vi "0x2 RIO-OCU update.vi"(11 "NetworkStreamWriter In":refnum<class "NetworkStreamWriter.lvclass">) -> (3 "NetworkStreamWriter Out":refnum<class "NetworkStreamWriter.lvclass">)   [LabVIEW 2011]
doc: "Sends general data up to the listening OCU over a network stream for monitoring and debugging purposes."
uses:
  0x2 Typedefs/RIO-OCU update controls.ctl
  2-Think/2 Typedefs/generalized sensor status.ctl
  2-Think/2 Typedefs/indicator LED.ctl
  2-Think/2 Typedefs/generalized actuator status.ctl
  2-Think/2 Typedefs/Which Boat.ctl
  2-Think/2 Typedefs/robot velocity.ctl
  2-Think/2 Typedefs/UTM Location.ctl
  2-Think/2 Typedefs/heading.ctl
  2-Think/2 Typedefs/rate of turn.ctl
  2-Think/2 Typedefs/pitch and roll.ctl
  2-Think/2 Typedefs/apparent wind.ctl
  2-Think/2 Typedefs/apparent wind speed.ctl
  2-Think/2 Typedefs/apparent wind direction.ctl
  2-Think/2 Typedefs/Velocity.ctl
  2-Think/2 Typedefs/absolute wind direction.ctl
  2-Think/2 Typedefs/absolute wind speed.ctl
  2-Think/2 Typedefs/absolute water current vector.ctl
  2-Think/2 Typedefs/rudder angle.ctl
  2-Think/2 Typedefs/sail setpt.ctl
  2-Think/2 Typedefs/manual override.ctl
  2-Think/2 Typedefs/setpoints to boat.ctl
  0x2 Typedefs/Waypoints List.ctl
  0x2 Typedefs/ocuWaypoint.ctl
  0x2 Typedefs/waypointTypes.ctl
  0x2 Typedefs/Current Waypoint.ctl
  0x2 Classes/NetworkStreams/Writer/NetworkStreamWriter.lvclass
  2-Think/2 Globals/2 Global.vi
panel:
  out "RIO->OCU update data":T1 {"Robot Pitch/Roll"."Roll" format="%05.1f"; "Robot Pitch/Roll"."Pitch" format="%05.1f"; "Robot\nRate of Turn" format="%05.1f"; "Robot\nHeading" format="%05.1f"}
  # "How Am I?"
  # "Where Am I?"
  # "Path Planning"
  # "From Planning Functions"
  # "(this is not a cluster because subitems\nare generated in parallel code)"
  # "What's Around Me?"
  # "As Measured"
  # "As Measured"
  # "Loop Rates"
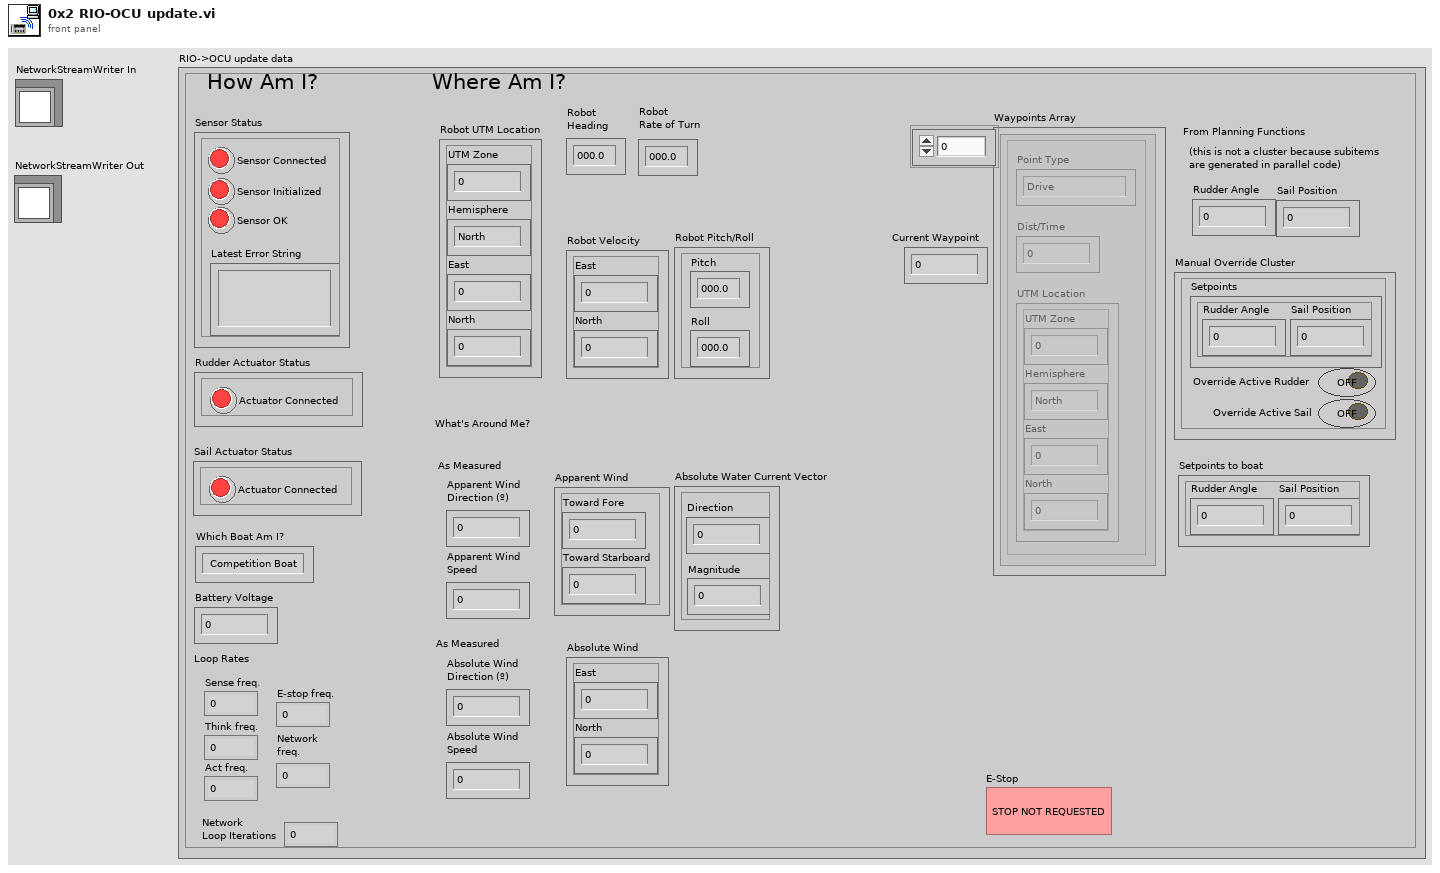
[diagram p1: front panel]
types:
  T1 = typedef "RIO-OCU update controls.ctl" = cluster{"Sensor Status":T2, "Battery Voltage":dbl, "Rudder Actuator Status":T4, "Sail Actuator Status":T4, "Which Boat Am I?":T5, "Robot Velocity":T6, "Robot UTM Location":T7, "Robot\nHeading ":T8, "Robot\nRate of Turn":T9, "Robot Pitch/Roll":T10, "Apparent Wind":T11, "Apparent Wind\nSpeed":T12, "Apparent Wind\nDirection (º)":T13, "Absolute Wind":T14, "Absolute Wind\nDirection (º)":T15, "Absolute Wind\nSpeed":T16, "Absolute Water Current Vector":T17, "Rudder Angle":T18, "Sail Position":T19, "Manual Override Cluster":T20, "Setpoints to boat":T21, "Waypoints Array":T22, "Current Waypoint":T25, "Think freq.":dbl, "Sense freq.":dbl, "Act freq.":dbl, "E-stop freq.":dbl, "Network \nfreq.":dbl, "Network \nLoop Iterations":i64, "E-Stop":bool}
  T2 = typedef "generalized sensor status.ctl" = cluster{"Sensor Connected":T3, "Sensor Initialized":T3, "Sensor OK":T3, "Latest Error String":string}
  T3 = typedef "indicator LED.ctl" = bool
  T4 = typedef "generalized actuator status.ctl" = cluster{"Actuator Connected":T3}
  T5 = typedef "Which Boat.ctl" = enum16{"Competition Boat", "Small RC", "Simulation"}
  T6 = typedef "robot velocity.ctl" = cluster{"East":dbl, "North":dbl}
  T7 = typedef "UTM Location.ctl" = cluster{"UTM Zone":dbl, "Hemisphere":enum16{"North", "South"}, "East":dbl, "North":dbl}
  T8 = typedef "heading.ctl" = dbl
  T9 = typedef "rate of turn.ctl" = dbl
  T10 = typedef "pitch and roll.ctl" = cluster{"Pitch":dbl, "Roll":dbl}
  T11 = typedef "apparent wind.ctl" = cluster{"Toward Fore":dbl, "Toward Starboard":dbl}
  T12 = typedef "apparent wind speed.ctl" = dbl
  T13 = typedef "apparent wind direction.ctl" = dbl
  T14 = typedef "Velocity.ctl" = cluster{"East":dbl, "North":dbl}
  T15 = typedef "absolute wind direction.ctl" = dbl
  T16 = typedef "absolute wind speed.ctl" = dbl
  T17 = typedef "absolute water current vector.ctl" = cluster{"Direction":T13, "Magnitude":T13}
  T18 = typedef "rudder angle.ctl" = dbl
  T19 = typedef "sail setpt.ctl" = dbl
  T20 = typedef "manual override.ctl" = cluster{"Override Active Rudder":bool, "Setpoints":T21, "Override Active Sail":bool}
  T21 = typedef "setpoints to boat.ctl" = cluster{"Sail Position":T19, "Rudder Angle":T18}
  T22 = typedef "Waypoints List.ctl" = T23[]
  T23 = typedef "ocuWaypoint.ctl" = cluster{"Point Type":T24, "Dist/Time":dbl, "UTM Location":T7}
  T24 = typedef "waypointTypes.ctl" = enum16{"Drive", "Round Port", "Round Starboard", "Stay"}
  T25 = typedef "Current Waypoint.ctl" = i32
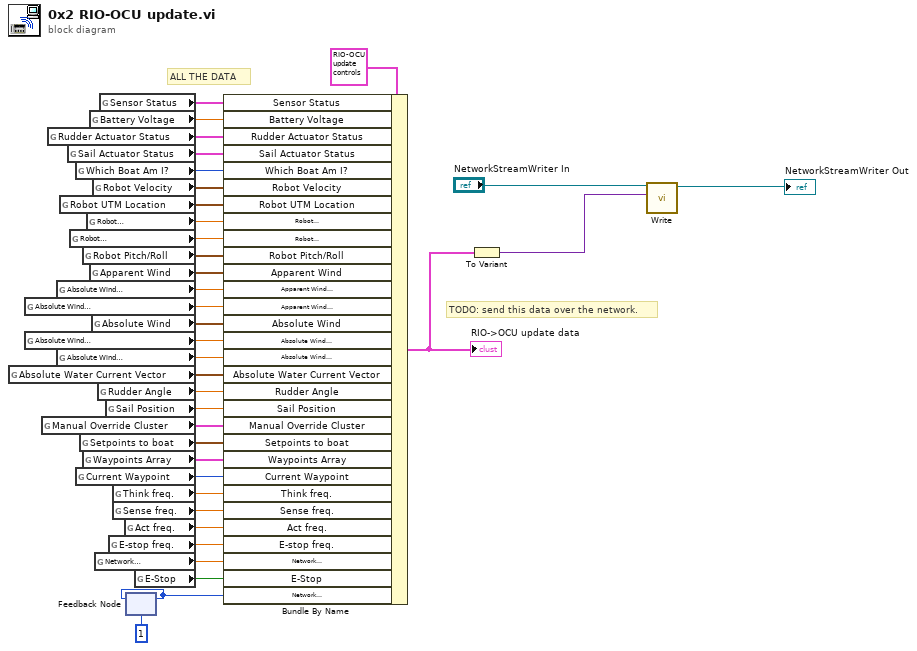
[diagram p0: block diagram]
diagram:
  # "ALL THE DATA"
  # "TODO: send this data over the network."
  n1 = global read "2 Global.vi" "Absolute Water Current Vector"() -> (w7:T17)
  n2 = global read "2 Global.vi" "Absolute Wind\nDirection (º)"() -> (w21:T15)
  n3 = global read "2 Global.vi" "Absolute Wind\nDirection (º)"() -> (w20:T15)
  n4 = global read "2 Global.vi" "Manual Override Cluster"() -> (w27:T20)
  n5 = global read "2 Global.vi" "Rudder Actuator Status"() -> (w14:T4)
  n6 = global read "2 Global.vi" "Absolute Wind\nSpeed"() -> (w22:T16)
  n7 = global read "2 Global.vi" "Absolute Wind\nSpeed"() -> (w19:T16)
  n8 = global read "2 Global.vi" "Robot UTM Location"() -> (w11:T7)
  n9 = global read "2 Global.vi" "Sail Actuator Status"() -> (w13:T4)
  n10 = global read "2 Global.vi" "Robot\nRate of Turn"() -> (w18:T9)
  n11 = global read "2 Global.vi" "Which Boat Am I?"() -> (w16:T5)
  n12 = global read "2 Global.vi" "Current Waypoint"() -> (w26:T25)
  n13 = global read "2 Global.vi" "Setpoints to boat"() -> (w24:T21)
  n14 = global read "2 Global.vi" "Robot Pitch/Roll"() -> (w10:T10)
  n15 = global read "2 Global.vi" "Waypoints Array"() -> (w25:T22)
  n16 = global read "2 Global.vi" "Robot\nHeading"() -> (w17:T8)
  n17 = global read "2 Global.vi" "Battery Voltage"() -> (w28:dbl)
  n18 = global read "2 Global.vi" "Apparent Wind"() -> (w9:T11)
  n19 = global read "2 Global.vi" "Absolute Wind"() -> (w8:T14)
  n20 = global read "2 Global.vi" "Robot Velocity"() -> (w12:T6)
  n21 = global read "2 Global.vi" "Network \nfreq."() -> (w31:dbl)
  n22 = global read "2 Global.vi" "Rudder Angle"() -> (w23:T18)
  n23 = global read "2 Global.vi" "Sensor Status"() -> (w15:T2)
  n24 = global read "2 Global.vi" "Sail Position"() -> (w29:T19)
  n25 = global read "2 Global.vi" "E-stop freq."() -> (w32:dbl)
  n26 = global read "2 Global.vi" "Think freq."() -> (w35:dbl)
  n27 = global read "2 Global.vi" "Sense freq."() -> (w34:dbl)
  n28 = global read "2 Global.vi" "Act freq."() -> (w33:dbl)
  n29 = feedback #1(i64 1) -> (w5:i64)
  n30 = feedback-in #1(w5) -> ()
  n31 = global read "2 Global.vi" "E-Stop"() -> (w30:bool)
  n32 = Bundle By Name(cluster=T1 {"Sensor Status"={"Sensor Connected"=FALSE, "Sensor Initialized"=FALSE, "Sensor OK"=FALSE, "Latest Error String"=""}, "Battery Voltage"=0.0, "Rudder Actuator Status"={"Actuator Connected"=FALSE}, "Sail Actuator Status"={"Actuator Connected"=FALSE}, "Which Boat Am I?"=enum."Competition Boat", "Robot Velocity"={"East"=0.0, "North"=0.0}, "Robot UTM Location"={"UTM Zone"=0.0, "Hemisphere"=enum."North", "East"=0.0, "North"=0.0}, "Robot\nHeading "=0.0, "Robot\nRate of Turn"=0.0, "Robot Pitch/Roll"={"Pitch"=0.0, "Roll"=0.0}, "Apparent Wind"={"Toward Fore"=0.0, "Toward Starboard"=0.0}, "Apparent Wind\nSpeed"=0.0, "Apparent Wind\nDirection (º)"=0.0, "Absolute Wind"={"East"=0.0, "North"=0.0}, "Absolute Wind\nDirection (º)"=0.0, "Absolute Wind\nSpeed"=0.0, "Absolute Water Current Vector"={"Direction"=0.0, "Magnitude"=0.0}, "Rudder Angle"=0.0, "Sail Position"=0.0, "Manual Override Cluster"={"Override Active Rudder"=FALSE, "Setpoints"={"Sail Position"=0.0, "Rudder Angle"=0.0}, "Override Active Sail"=FALSE}, "Setpoints to boat"={"Sail Position"=0.0, "Rudder Angle"=0.0}, "Waypoints Array"=[], "Current Waypoint"=0, "Think freq."=0.0, "Sense freq."=0.0, "Act freq."=0.0, "E-stop freq."=0.0, "Network \nfreq."=0.0, "Network \nLoop Iterations"=0, "E-Stop"=FALSE} ("Monitored Items from RIO"), "Sensor Status"=w15, "Battery Voltage"=w28, "Rudder Actuator Status"=w14, "Sail Actuator Status"=w13, "Which Boat Am I?"=w16, "Robot Velocity"=w12, "Robot UTM Location"=w11, "Robot\nHeading"=w17, "Robot\nRate of Turn"=w18, "Robot Pitch/Roll"=w10, "Apparent Wind"=w9, "Apparent Wind\nSpeed"=w22, "Apparent Wind\nDirection (º)"=w21, "Absolute Wind"=w8, "Absolute Wind\nDirection (º)"=w20, "Absolute Wind\nSpeed"=w19, "Absolute Water Current Vector"=w7, "Rudder Angle"=w23, "Sail Position"=w29, "Manual Override Cluster"=w27, "Setpoints to boat"=w24, "Waypoints Array"=w25, "Current Waypoint"=w26, "Think freq."=w35, "Sense freq."=w34, "Act freq."=w33, "E-stop freq."=w32, "Network \nfreq."=w31, "E-Stop"=w30, "Network \nLoop Iterations"=w5) -> (w2:T1)
  "RIO->OCU update data" <- w2
  n33 = To Variant(anything=w2) -> (Variant=w1:variant)
  n34 = call "Write.vi"("element"=w1, "NetworkStreamWriter in"="NetworkStreamWriter In") -> ("NetworkStreamWriter out"=→"NetworkStreamWriter Out":refnum<class "NetworkStreamWriter.lvclass">)  [unwired: 8 in, 1 out]
